vi "GIF.Read.Unpack.State__ogtk.vi"(6 "error in (no error)":errorcluster, 8 "ColorMap":bool, 9 "NextLabel":u8, 10 "NextCharacter":u8, 11 "State in":T1(ring)=enum."End_Of_File") -> (3 "New State":T1(ring)=enum."End_Of_File", 4 "error out":errorcluster)   [LabVIEW 2018]
panel:
  # "GIF.Read.Unpack.State.vi\n\nGoverns state-transitions for GIF.Read.Unpackvi\n\nPlease visit http://www.OpenG.org to learn about the\nOpen Source LabVIEW software movement.\n\nNOTICE -- YOU MUST LEAVE THIS NOTICE IN PLACE.  PER THE TERMS OF THE LICENSE BELOW, YOU MAY SUBLICENSE THIS SOFTWARE \nIN ANY WAY THAT DOES NOT CONFLICT WITH THIS LICENSE.\n\n### BSD License (http://www.opensource.org/licenses/bsd-license.php) Begin ###\n \nCopyright (c) 2007, Bill Clench <bclench@yahoo.com>\n\nAll rights reserved.\n\nRedistribution and use in source and binary forms, with or without modification, are permitted provided that the following conditions are met:\n\n    * Redistributions of source code must retain the above copyright notice, this list of conditions and the following disclaimer.\n    * Redistributions in binary form must reproduce the above copyright notice, this list of conditions and the following disclaimer in the \n       documentation and/or other materials provided with the distribution.\n    * Neither the name of SciWare, James Kring, Inc., nor the names of its contributors may be used to endorse or promote products derived \n       from this software without specific prior written permission.\n\nTHIS SOFTWARE IS PROVIDED BY THE COPYRIGHT HOLDERS AND CONTRIBUTORS \"AS IS\" AND ANY EXPRESS OR IMPLIED WARRANTIES, \nINCLUDING, BUT NOT LIMITED TO, THE IMPLIED WARRANTIES OF MERCHANTABILITY AND FITNESS FOR A PARTICULAR PURPOSE ARE \nDISCLAIMED. IN NO EVENT SHALL THE COPYRIGHT OWNER OR CONTRIBUTORS BE LIABLE FOR ANY DIRECT, INDIRECT, INCIDENTAL,\n SPECIAL, EXEMPLARY, OR CONSEQUENTIAL DAMAGES (INCLUDING, BUT NOT LIMITED TO, PROCUREMENT OF SUBSTITUTE GOODS OR \nSERVICES; LOSS OF USE, DATA, OR PROFITS; OR BUSINESS INTERRUPTION) HOWEVER CAUSED AND ON ANY THEORY OF LIABILITY, \nWHETHER IN CONTRACT, STRICT LIABILITY, OR TORT (INCLUDING NEGLIGENCE OR OTHERWISE) ARISING IN ANY WAY OUT OF THE USE \nOF THIS SOFTWARE, EVEN IF ADVISED OF THE POSSIBILITY OF SUCH DAMAGE.\n\n### BSD License End ###"
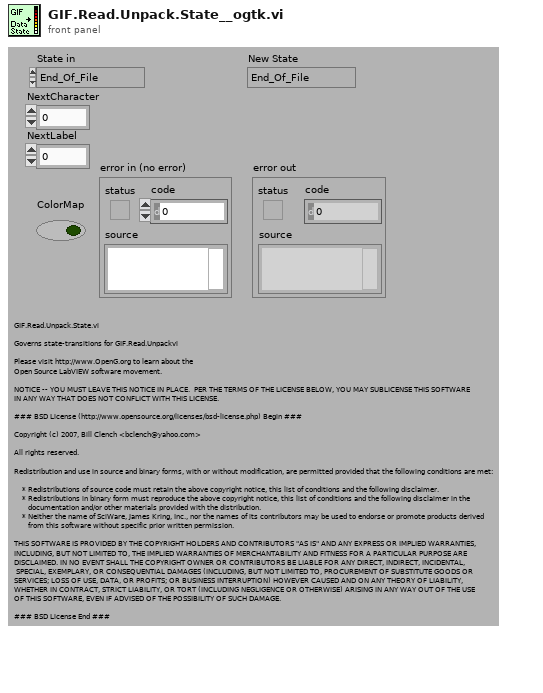
[diagram p1: front panel]
types:
  T1 = enum16{"Begin", "Header", "LS_LSDescriptor", "LS_GCTable", "Data_LGD_SPB", "Data_GB_GRB_PTE", "Data_GB_GCE", "Data_GB_GRB_TBI_IDesc", "Data_GB_GRB_TBI_CMap", "Data_GB_GRB_TBI_ImageData", "End_Of_File"}
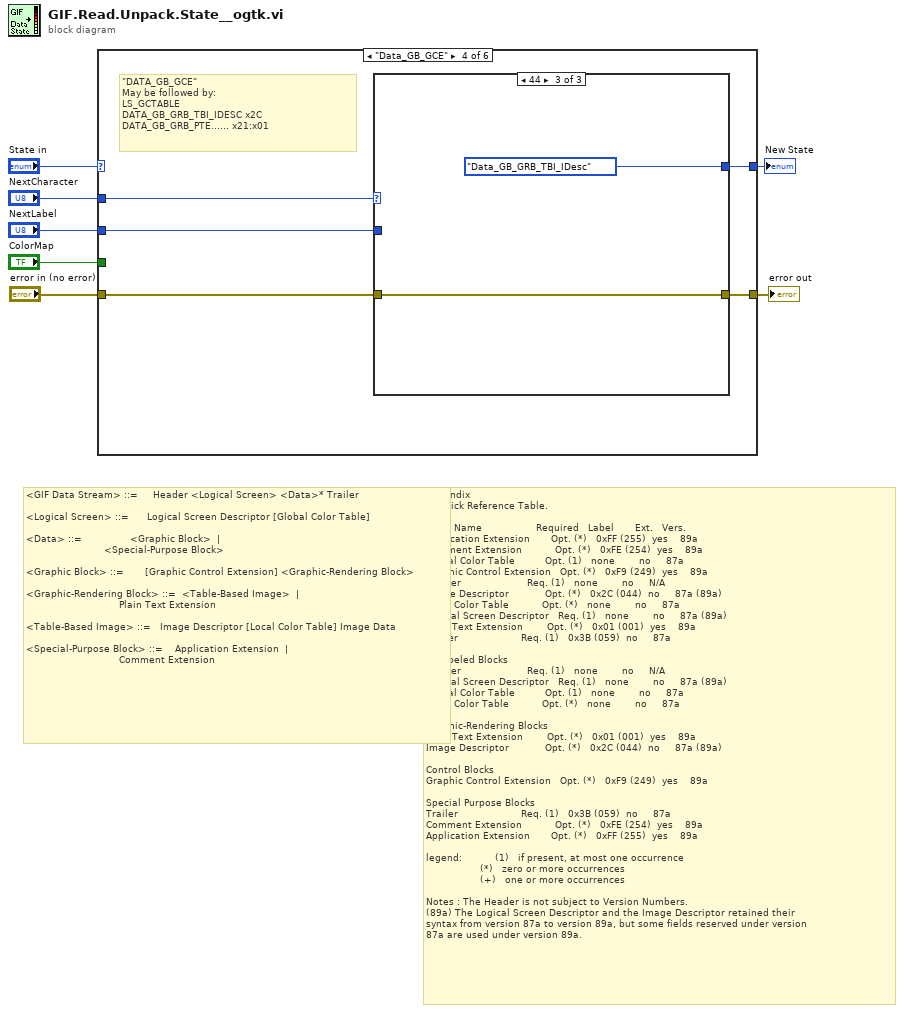
[diagram p0: block diagram]
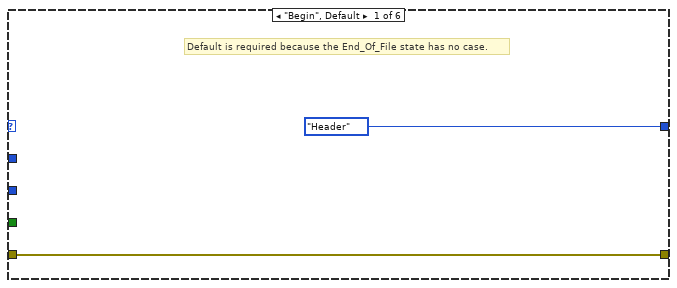
[diagram p2: hidden frame]
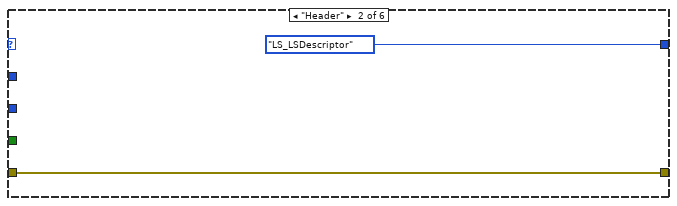
[diagram p3: hidden frame]
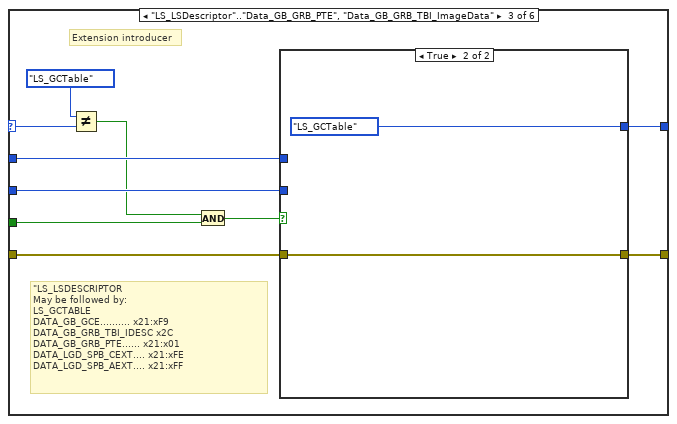
[diagram p4: hidden frame]
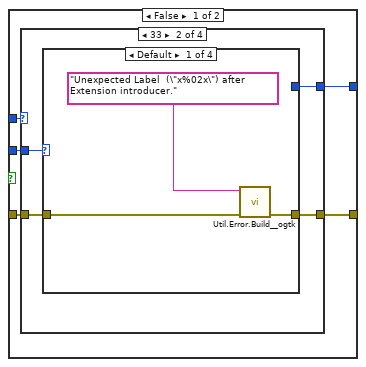
[diagram p5: hidden frame]
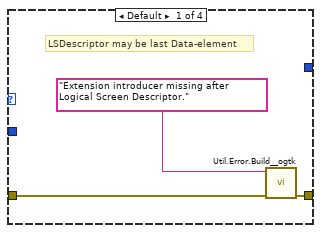
[diagram p6: hidden frame]
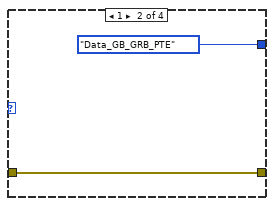
[diagram p7: hidden frame]
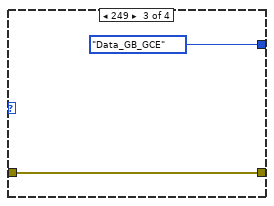
[diagram p8: hidden frame]
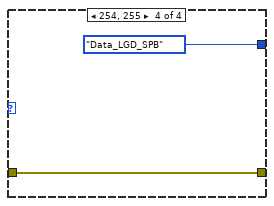
[diagram p9: hidden frame]
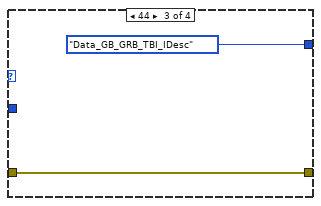
[diagram p10: hidden frame]
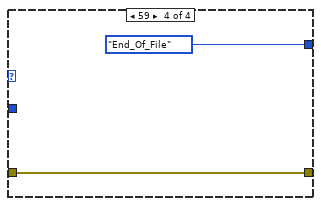
[diagram p11: hidden frame]
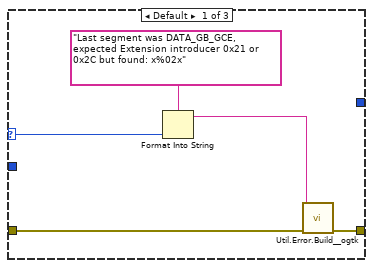
[diagram p12: hidden frame]
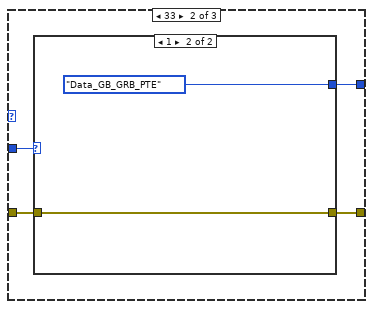
[diagram p13: hidden frame]
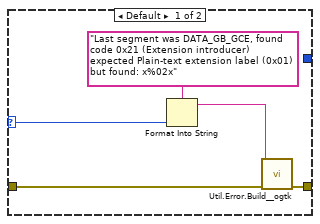
[diagram p14: hidden frame]
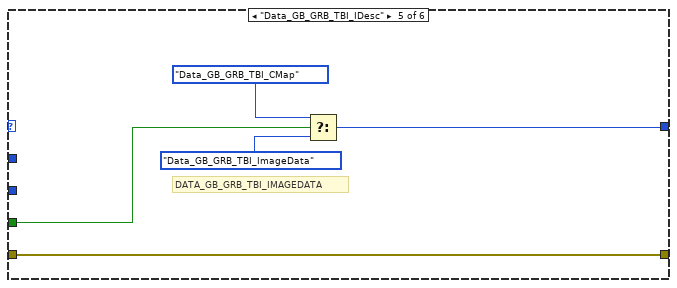
[diagram p15: hidden frame]
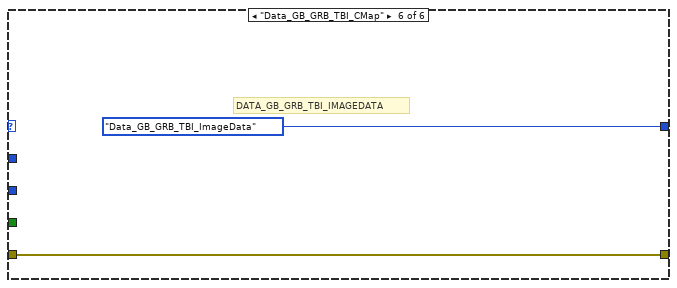
[diagram p16: hidden frame]
diagram:
  # "Appendix\nA. Quick Reference Table.\n\nBlock Name                  Required   Label       Ext.   Vers.\nApplication Extension       Opt. (*)   0xFF (255)  yes    89a\nComment Extension           Opt. (*)   0xFE (254)  yes    89a\nGlobal Color Table          Opt. (1)   none        no     87a\nGraphic Control Extension   Opt. (*)   0xF9 (249)  yes    89a\nHeader                      Req. (1)   none        no     N/A\nImage Descriptor            Opt. (*)   0x2C (044)  no     87a (89a)\nLocal Color Table           Opt. (*)   none        no     87a\nLogical Screen Descriptor   Req. (1)   none        no     87a (89a)\nPlain Text Extension        Opt. (*)   0x01 (001)  yes    89a\nTrailer                     Req. (1)   0x3B (059)  no     87a\n\nUnlabeled Blocks\nHeader                      Req. (1)   none        no     N/A\nLogical Screen Descriptor   Req. (1)   none        no     87a (89a)\nGlobal Color Table          Opt. (1)   none        no     87a\nLocal Color Table           Opt. (*)   none        no     87a\n\nGraphic-Rendering Blocks\nPlain Text Extension        Opt. (*)   0x01 (001)  yes    89a\nImage Descriptor            Opt. (*)   0x2C (044)  no     87a (89a)\n\nControl Blocks\nGraphic Control Extension   Opt. (*)   0xF9 (249)  yes    89a\n\nSpecial Purpose Blocks\nTrailer                     Req. (1)   0x3B (059)  no     87a\nComment Extension           Opt. (*)   0xFE (254)  yes    89a\nApplication Extension       Opt. (*)   0xFF (255)  yes    89a\n\nlegend:           (1)   if present, at most one occurrence\n                  (*)   zero or more occurrences\n                  (+)   one or more occurrences\n\nNotes : The Header is not subject to Version Numbers.\n(89a) The Logical Screen Descriptor and the Image Descriptor retained their\nsyntax from version 87a to version 89a, but some fields reserved under version\n87a are used under version 89a."
  # "<GIF Data Stream> ::=     Header <Logical Screen> <Data>* Trailer\n\n<Logical Screen> ::=      Logical Screen Descriptor [Global Color Table]\n\n<Data> ::=                <Graphic Block>  |\n                          <Special-Purpose Block>\n\n<Graphic Block> ::=       [Graphic Control Extension] <Graphic-Rendering Block>\n\n<Graphic-Rendering Block> ::=  <Table-Based Image>  |\n                               Plain Text Extension\n\n<Table-Based Image> ::=   Image Descriptor [Local Color Table] Image Data\n\n<Special-Purpose Block> ::=    Application Extension  |\n                               Comment Extension"
  n1 = case shown="\"Data_GB_GCE\"" "State in" {
    selector: "State in" -> [_ _ w16 _ _ _]
    tunnel: [T1."Header" ("State") T1."LS_LSDescriptor" ("State") w21 w49 w75 T1."Data_GB_GRB_TBI_ImageData" ("State")] -> w6
    tunnel: "NextCharacter" -> [_ _ w20 w53 _ _]
    tunnel: "NextLabel" -> [_ _ w19 w52 _ _]
    tunnel: "ColorMap" -> [_ _ w15 _ w76 _]
    tunnel: "error in (no error)" -> [w9 w11 w18 w51 w74 w78]
    tunnel: [w9 w11 w17 w50 w74 w78] -> w1
    frame "Begin", Default {
      # "Default is required because the End_Of_File state has no case."
    }
    frame "Header" {
    }
    frame "LS_LSDescriptor".."Data_GB_GRB_PTE", "Data_GB_GRB_TBI_ImageData" {
      # "Extension introducer"
      # "\"LS_LSDESCRIPTOR \nMay be followed by:\nLS_GCTABLE\nDATA_GB_GCE.......... x21:xF9\nDATA_GB_GRB_TBI_IDESC x2C\nDATA_GB_GRB_PTE...... x21:x01\nDATA_LGD_SPB_CEXT.... x21:xFE\nDATA_LGD_SPB_AEXT.... x21:xFF"
      n2 = Not Equal?(x=T1."LS_GCTable" ("State"), y=w16) -> (x != y?=w14:bool)
      n3 = And(x=w14, y=w15) -> (x .and. y?=w13:bool)
      n4 = case shown="True" w13 {
        tunnel: [w26 T1."LS_GCTable" ("State")] -> w21
        tunnel: w20 -> [w25 _]
        tunnel: w19 -> [w24 _]
        tunnel: w18 -> [w23 w48]
        tunnel: [w22 w48] -> w17
        frame False {
          n5 = case shown="33" w25 {
            tunnel: [_ w33 T1."Data_GB_GRB_TBI_IDesc" ("State") T1."End_Of_File" ("State")] -> w26
            tunnel: w24 -> [_ w32 _ _]
            tunnel: w23 -> [w28 w31 w44 w46]
            tunnel: [w29 w30 w44 w46] -> w22
            frame Default {
              # "LSDescriptor may be last Data-element"
              n6 = call <userlib>:"Util.Error.Build__ogtk.vi"("error in (no error)"=w28, "Source"="Extension introducer missing after Logical Screen Descriptor.") -> ("error out"=w29:errorcluster)  [unwired: 9 in]
            }
            frame 33 {
              n7 = case shown="Default" w32 {
                tunnel: [_ T1."Data_GB_GRB_PTE" ("State") T1."Data_GB_GCE" ("State") T1."Data_LGD_SPB" ("State")] -> w33
                tunnel: w31 -> [w35 w38 w40 w42]
                tunnel: [w36 w38 w40 w42] -> w30
                frame Default {
                  n8 = call <userlib>:"Util.Error.Build__ogtk.vi"("error in (no error)"=w35, "Source"="Unexpected Label  (\"x%02x\") after Extension introducer.") -> ("error out"=w36:errorcluster)  [unwired: 9 in]
                }
                frame 1 {
                }
                frame 249 {
                }
                frame 254, 255 {
                }
              }
            }
            frame 44 {
            }
            frame 59 {
            }
          }
        }
        frame True {
        }
      }
    }
    frame "Data_GB_GCE" {
      # "\"DATA_GB_GCE\"\nMay be followed by:\nLS_GCTABLE\nDATA_GB_GRB_TBI_IDESC x2C\nDATA_GB_GRB_PTE...... x21:x01"
      n9 = case shown="44" w53 {
        selector: w53 -> [w57 _ _]
        tunnel: w52 -> [_ w62 _]
        tunnel: w51 -> [w56 w61 w71]
        tunnel: [w55 w60 w71] -> w50
        tunnel: [_ w59 T1."Data_GB_GRB_TBI_IDesc" ("State")] -> w49
        frame Default {
          n10 = Format Into String(format string="Last segment was DATA_GB_GCE, expected Extension introducer 0x21 or 0x2C but found: x%02x", w57) -> (resulting string=w54:string)  [unwired: 2 in, 1 out]
          n11 = call <userlib>:"Util.Error.Build__ogtk.vi"("error in (no error)"=w56, "Source"=w54) -> ("error out"=w55:errorcluster)  [unwired: 9 in]
        }
        frame 33 {
          n12 = case shown="1" w62 {
            selector: w62 -> [w67 _]
            tunnel: w61 -> [w65 w69]
            tunnel: [w64 w69] -> w60
            tunnel: [_ T1."Data_GB_GRB_PTE" ("State")] -> w59
            frame Default {
              n13 = Format Into String(format string="Last segment was DATA_GB_GCE, found code 0x21 (Extension introducer) expected Plain-text extension label (0x01) but found: x%02x", w67) -> (resulting string=w63:string)  [unwired: 2 in, 1 out]
              n14 = call <userlib>:"Util.Error.Build__ogtk.vi"("error in (no error)"=w65, "Source"=w63) -> ("error out"=w64:errorcluster)  [unwired: 9 in]
            }
            frame 1 {
            }
          }
        }
        frame 44 {
        }
      }
    }
    frame "Data_GB_GRB_TBI_IDesc" {
      # "DATA_GB_GRB_TBI_IMAGEDATA"
      n15 = Select(t=T1."Data_GB_GRB_TBI_CMap" ("State"), s=w76, f=T1."Data_GB_GRB_TBI_ImageData" ("State")) -> (s? t:f=w75:T1)
    }
    frame "Data_GB_GRB_TBI_CMap" {
      # "DATA_GB_GRB_TBI_IMAGEDATA"
    }
  }
  "New State" <- w6
  "error out" <- w1
